vi "SelectStriptestProber.vi"(8 "error in (no error)":errorcluster) -> (0 "error out":errorcluster, 3 "ProbeStationControl out":refnum<class "ProbeStationControl.lvclass">)   [LabVIEW 2019, in "ProbeStationControl.lvclass"]
uses:
  ProbeStationControl.lvclass
  Alessi Rel-6100/AlessiRel6100.lvclass
  C:/Users/Semiprobe/Desktop/Probe-Test-Software/itk-strip-sensor-qc/LabVIEW 2019/InstrControl/ProbeStationControl/ProbeStationControl.lvclass
  SemiProbe/SemiProbe.lvclass
panel:
  out "Tab Control":enum32{"Select Prober"}(tab)
  in  "Select Probestation":enum16{"Alessi REL-6100", "SemiProbe"}(ring)
  in  "Cancel Button":bool
  in  "Continue":bool
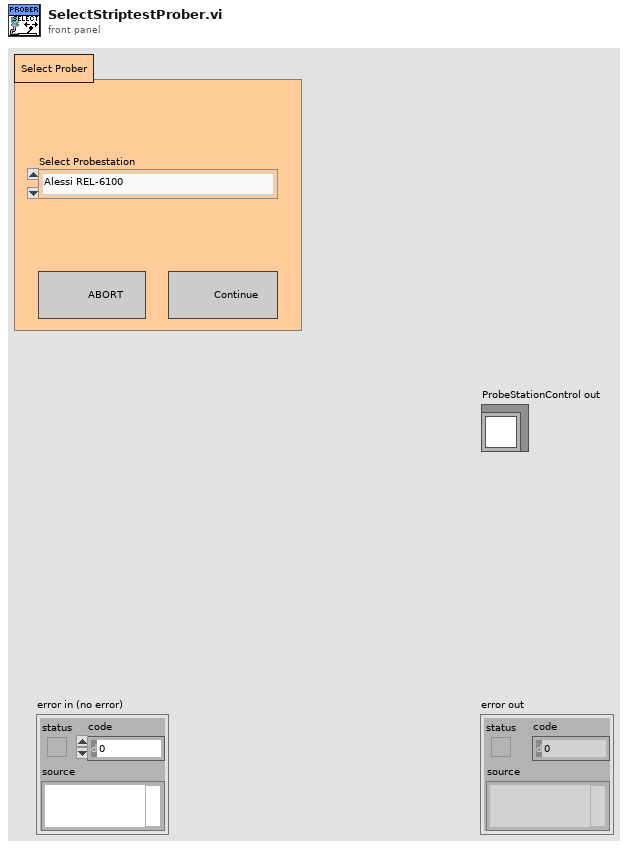
[diagram p1: front panel]
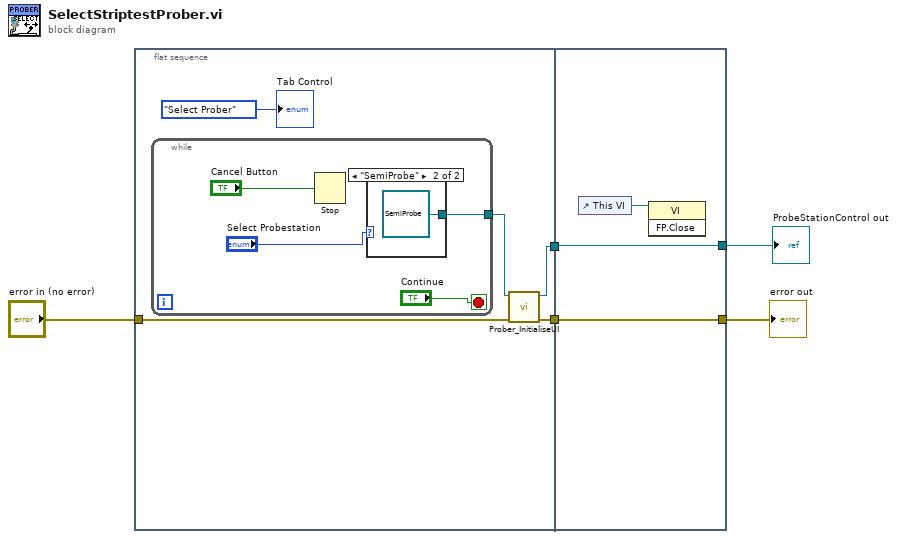
[diagram p0: block diagram]
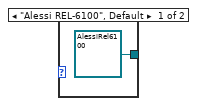
[diagram p2: hidden frame]
diagram:
  n1 = flat-sequence {
    tunnel: "error in (no error)" -> [w8]
    tunnel: [w7] -> w2
    tunnel: [w6] -> w1
    tunnel: [w18] -> w3
    tunnel: [w17] -> w4
    tunnel: w2 -> [w18]
    tunnel: w1 -> [w17]
    frame #0 {
      n2 = while {
        tunnel: [w11] -> w9
        stop <- "Continue" stop-if-true
        n3 = Stop(stop? (T)="Cancel Button") -> ()
        n4 = case shown="\"SemiProbe\"" "Select Probestation" {
          tunnel: [refnum<class "AlessiRel6100.lvclass"> refnum ("AlessiRel6100.lvclass") refnum<class "SemiProbe.lvclass"> refnum ("SemiProbe.lvclass")] -> w11
          frame "Alessi REL-6100", Default {
          }
          frame "SemiProbe" {
          }
        }
      }
      n5 = call-dynamic "Prober_InitialiseUI.vi"("error in (no error)"=w8, "ProbeStationControl in"=w9) -> ("error out"=w6:errorcluster, "ProbeStationControl out"=w7:refnum<class "ProbeStationControl.lvclass">)  [unwired: 7 in, 1 out]
      "Tab Control" <- enum32{"Select Prober", "Load sensor"}."Select Prober" ("Tab Control")
    }
    frame #1 {
      n6 = control-ref of="This VI"() -> (w19:refnum<vi>)
      n7 = invoke class="VI" method="FP.Close"(reference=w19) -> ()  [unwired: 2 in, 3 out]
    }
  }
  "ProbeStationControl out" <- w3
  "error out" <- w4
